vi "Generate Error Cluster.vi"(9 "Error active?":bool, 11 "Error_message":string) -> (0 "error out":errorcluster)   [LabVIEW 2016, in "Environment Chamber.lvlib" / "Climatic Chamber.lvlib"]
uses:
  Climatic Chamber.lvlib
  <vilib>/Utility/error.llb/DialogType.ctl
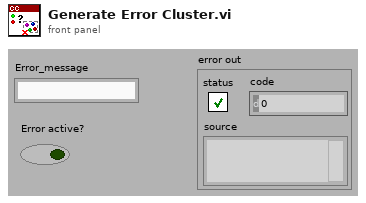
[diagram p1: front panel]
types:
  T1 = typedef "DialogType.ctl" = u16
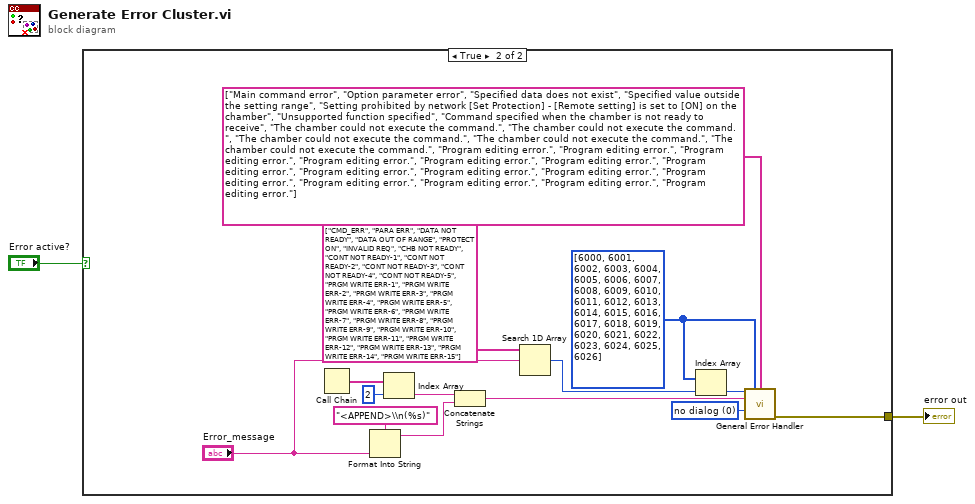
[diagram p0: block diagram]
diagram:
  n1 = case shown="True" "Error active?" {
    tunnel: [_ w3] -> w2
    frame False {
    }
    frame True {
      w15 = T1 0 items=["no dialog", "OK message", "continue or stop message", "OK message + warnings", "continue/stop + warnings"] ("type of dialog (OK msg:1)")
      w7 = i32[] [6000, 6001, 6002, 6003, 6004, 6005, 6006, 6007, 6008, 6009, 6010, 6011, 6012, 6013, 6014, 6015, 6016, 6017, 6018, 6019, 6020, 6021, 6022, 6023, 6024, 6025, 6026] ("[user-defined codes]")
      n2 = Call Chain() -> (call chain=w14:string[])
      n3 = Format Into String(format string="<APPEND>\\n(%s)", "Error_message") -> (resulting string=w10:string)  [unwired: 2 in, 1 out]
      n4 = Index Array(array=w14, index=2) -> (element=w12:string)
      n5 = Concatenate Strings(w12, w10) -> (w4:string)
      n6 = Search 1D Array(1D array=string[] ["CMD_ERR", "PARA ERR", "DATA NOT READY", "DATA OUT OF RANGE", "PROTECT ON", "INVALID REQ", "CHB NOT READY", "CONT NOT READY-1", "CONT NOT READY-2", "CONT NOT READY-3", "CONT NOT READY-4", "CONT NOT READY-5", "PRGM WRITE ERR-1", "PRGM WRITE ERR-2", "PRGM WRITE ERR-3", "PRGM WRITE ERR-4", "PRGM WRITE ERR-5", "PRGM WRITE ERR-6", "PRGM WRITE ERR-7", "PRGM WRITE ERR-8", "PRGM WRITE ERR-9", "PRGM WRITE ERR-10", "PRGM WRITE ERR-11", "PRGM WRITE ERR-12", "PRGM WRITE ERR-13", "PRGM WRITE ERR-14", "PRGM WRITE ERR-15"], element="Error_message") -> (index of element=w8:i32)  [unwired: 1 in]
      n7 = Index Array(array=w7, index=w8) -> (element=w6:i32)
      n8 = call <vilib>:"General Error Handler.vi"("[error code] (0)"=w6, "[user-defined codes]"=w7, "[user-defined descriptions]"=string[] ["Main command error", "Option parameter error", "Specified data does not exist", "Specified value outside the setting range", "Setting prohibited by network [Set Protection] - [Remote setting] is set to [ON] on the chamber", "Unsupported function specified", "Command specified when the chamber is not ready to receive", "The chamber could not execute the command.", "The chamber could not execute the command.", "The chamber could not execute the command.", "The chamber could not execute the command.", "The chamber could not execute the command.", "Program editing error.", "Program editing error.", "Program editing error.", "Program editing error.", "Program editing error.", "Program editing error.", "Program editing error.", "Program editing error.", "Program editing error.", "Program editing error.", "Program editing error.", "Program editing error.", "Program editing error.", "Program editing error.", "Program editing error."], "[error source] (\" \")"=w4, "type of dialog (OK msg:1)"=w15) -> ("error out"=w3:errorcluster)  [unwired: 6 in, 4 out]
    }
  }
  "error out" <- w2
